vi "f43.vi"() -> ()   [LabVIEW 2014]
panel:
  in  "f43":dbl
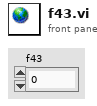
[diagram p1: front panel]
diagram:
